vi "ep_Butterworth Filter.vi"(4 "init/cont (init:F)":bool, 6 "order":i32=2, 7 "filter type":T1, 8 "low cutoff freq: fl":dbl=0.12500000000000006 format="%0.4f", 9 "high cutoff freq: fh":dbl=0.45000000000000007 format="%0.2f", 10 "sampling freq: fs":dbl=1.0 format="%0.2f", 11 "X":dbl[](array[numeric])) -> (0 "error":i32, 3 "Filtered X":dbl[](array[numeric]))   [LabVIEW 2011, in "NI_EP_Power Quality.lvlib"]
uses:
  <vilib>/Analysis/3filter.llb/Filter Passband Type.ctl
  <vilib>/Analysis/baseanly.llb/IIR Cascade Filter (DBL).vi
  <vilib>/addons/Electrical Power/PQ/NI_EP_Power Quality.lvlib
  <vilib>/Analysis/NI_AALBase.lvlib
panel:
  # "Butterworth Filter"
  # "Filter Controls"
  # "Frequency Controls"
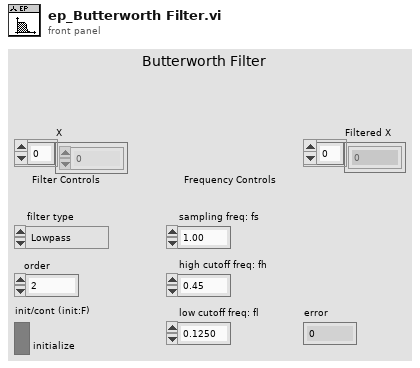
[diagram p1: front panel]
types:
  T1 = typedef "NI_AALBase.lvlib/Filter Passband Type.ctl" = enum32{"Lowpass", "Highpass", "Bandpass", "Bandstop"}
  T2 = cluster{"filter structure":enum32{"IIR 2nd Order", "IIR 4th Order"}, "Reverse Coefficients":dbl[], "Forward Coefficients":dbl[]}
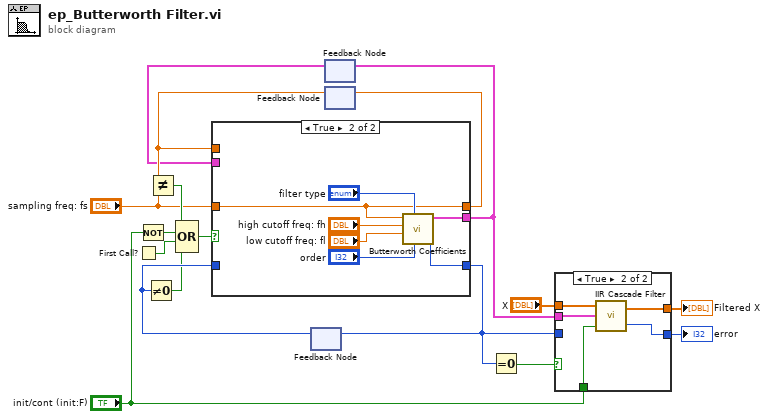
[diagram p0: block diagram]
diagram:
  n1 = First Call?() -> (First Call?: T/F=w10:bool)
  n2 = Not(x="init/cont (init:F)") -> (.not. x?=w9:bool)
  n3 = feedback #1() -> (w17:i32)  [unwired: 1 in]
  n4 = Not Equal To 0?(x=w17) -> (x != 0?=w16:bool)
  n5 = feedback #2() -> (w5:T2)  [unwired: 1 in]
  n6 = feedback #3() -> (w15:dbl)  [unwired: 1 in]
  n7 = Not Equal?(x=w15, y="sampling freq: fs") -> (x != y?=w14:bool)
  n8 = Compound Arithmetic op=OR(w14, w9, w10, w16) -> (w7:bool)
  n9 = case shown="True" w7 {
    tunnel: [w20 w24] -> w11
    tunnel: [w19 w21] -> w6
    tunnel: w5 -> [w20 _]
    tunnel: w17 -> [w19 _]
    tunnel: [w18 w22] -> w12
    tunnel: "sampling freq: fs" -> [_ w22]
    tunnel: w15 -> [w18 _]
    frame False {
    }
    frame True {
      n10 = call <vilib>:"Butterworth Coefficients.vi"("order"="order", "filter type"="filter type", "low cutoff freq: fl"="low cutoff freq: fl", "high cutoff freq: fh"="high cutoff freq: fh", "sampling freq: fs"=w22) -> ("error"=w21:i32, "IIR Filter Cluster"=w24:T2)  [unwired: 5 in]
    }
  }
  n11 = feedback-in #1(w6) -> ()
  n12 = feedback-in #2(w11) -> ()
  n13 = feedback-in #3(w12) -> ()
  n14 = Equal To 0?(x=w6) -> (x = 0?=w4:bool)
  n15 = case shown="True" w4 {
    tunnel: w6 -> [w28 _]
    tunnel: "X" -> [_ w33]
    tunnel: [_ w30] -> w2
    tunnel: w11 -> [_ w32]
    tunnel: [w28 w31] -> w3
    tunnel: "init/cont (init:F)" -> [_ w29]
    frame False {
    }
    frame True {
      n16 = call-poly <vilib>:"IIR Cascade Filter.vi"("init/cont (init:F)"=w29, "IIR Filter Cluster"=w32, "X"=w33) -> ("error"=w31:i32, "Filtered X"=w30:dbl[])
    }
  }
  "Filtered X" <- w2
  "error" <- w3
